vi "Stereo - Calibration Manager.vi"(7 "Function":T5, 10 "Right Grid Image":cluster{"Grid Image":T1, "Reference Points":T3}, 11 "Left Grid Image":cluster{"Grid Image":T1, "Reference Points":T3}) -> (0 "Calibration OK":bool, 1 "Calibrated Images":T1[](array[typedef]), 2 "Grid Coverage":T2, 3 "Grid Images out":cluster{"Left Image":T1, "Right Image":T1}[](array[cluster]))   [LabVIEW 2019]
doc: "Keeps track of the calibration grids needed to calibrate each camera.\nComputes the left and right camera models needed to compute the stereo calibration."
uses:
  Stereo - Calibration Manager Function.ctl
  <vilib>/vision/Image Controls.llb/IMAQ Image.ctl
  <vilib>/vision/Calibration.llb/Calibration Reference Points.ctl
  <vilib>/vision/Image Controls.llb/Vision Info Type2.ctl
  <vilib>/vision/NI_Vision_Development_Module.lvlib
panel:
  # "Overview: Keeps track of the calibration grids needed to calibrate each camera.\n                    Computes the left and right camera models needed to compute the stereo calibration."
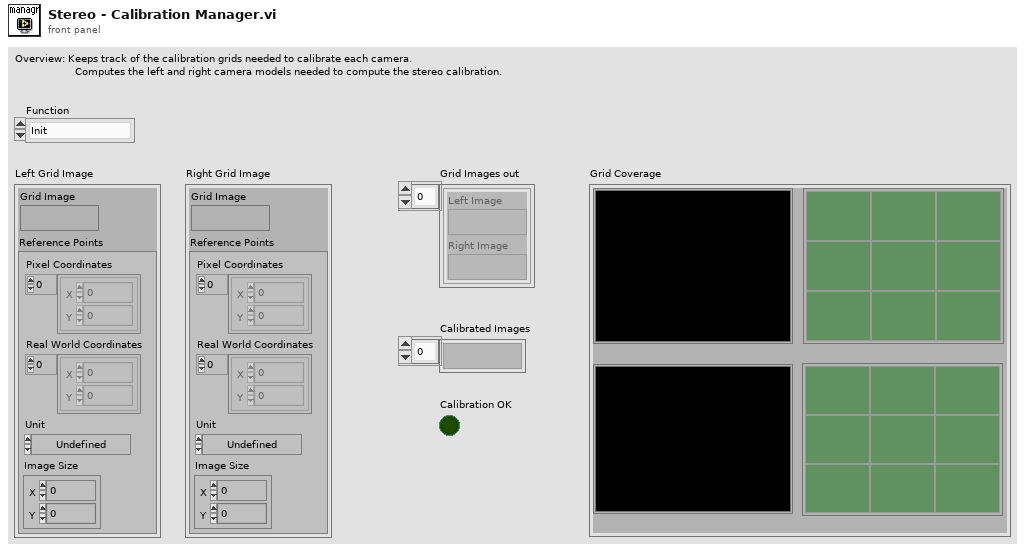
[diagram p1: front panel]
types:
  T1 = typedef "IMAQ Image.ctl" = refnum<image>
  T2 = cluster{"Left Image":T1, "Left Grid Coverage":bool[][], "Left Grid Coverage 3":string[][], "Right Image":T1, "Left Grid Coverage 2":bool[][], "Left Grid Coverage 4":string[][]}
  T3 = typedef "Calibration Reference Points.ctl" = cluster{"Pixel Coordinates":cluster{"X":dbl, "Y":dbl}[], "Real World Coordinates":cluster{"X":dbl, "Y":dbl}[], "Unit":T4, "Image Size":cluster{"X":u32, "Y":u32}}
  T4 = typedef "Image Unit" = enum32{"Undefined", "Angström", "Micrometer", "Millimeter", "Centimeter", "Meter", "Kilometer", "Microinch", "Inch", "Feet", "Nautical miles", "Standard miles", "Steps"}
  T5 = typedef "Stereo - Calibration Manager Function.ctl" = enum16{"Init", "Add Grid Images", "Get Images", "Dispose"}
  T6 = cluster{"Image Dst Out":T1, "Reference Points":T3}[][]
  T7 = cluster{"Left Image":T1, "Left Quadrants Status":bool[][], "Left Grid Coverage":string[][], "Right Image":T1, "Right Quadrant Status":bool[][], "Right Grid Coverage":string[][]}
  T8 = typedef "Vision Info Type2.ctl" = u32
  T9 = cluster{"Grid Image":T1, "Reference Points":T3}[]
  T10 = cluster{"Image Dst Out":T1, "Reference Points":T3}[]
  T11 = cluster{"Image Dst Out":T1, "Reference Points":T3}
  T12 = cluster{"Grid Image":T1, "Reference Points":T3}[][]
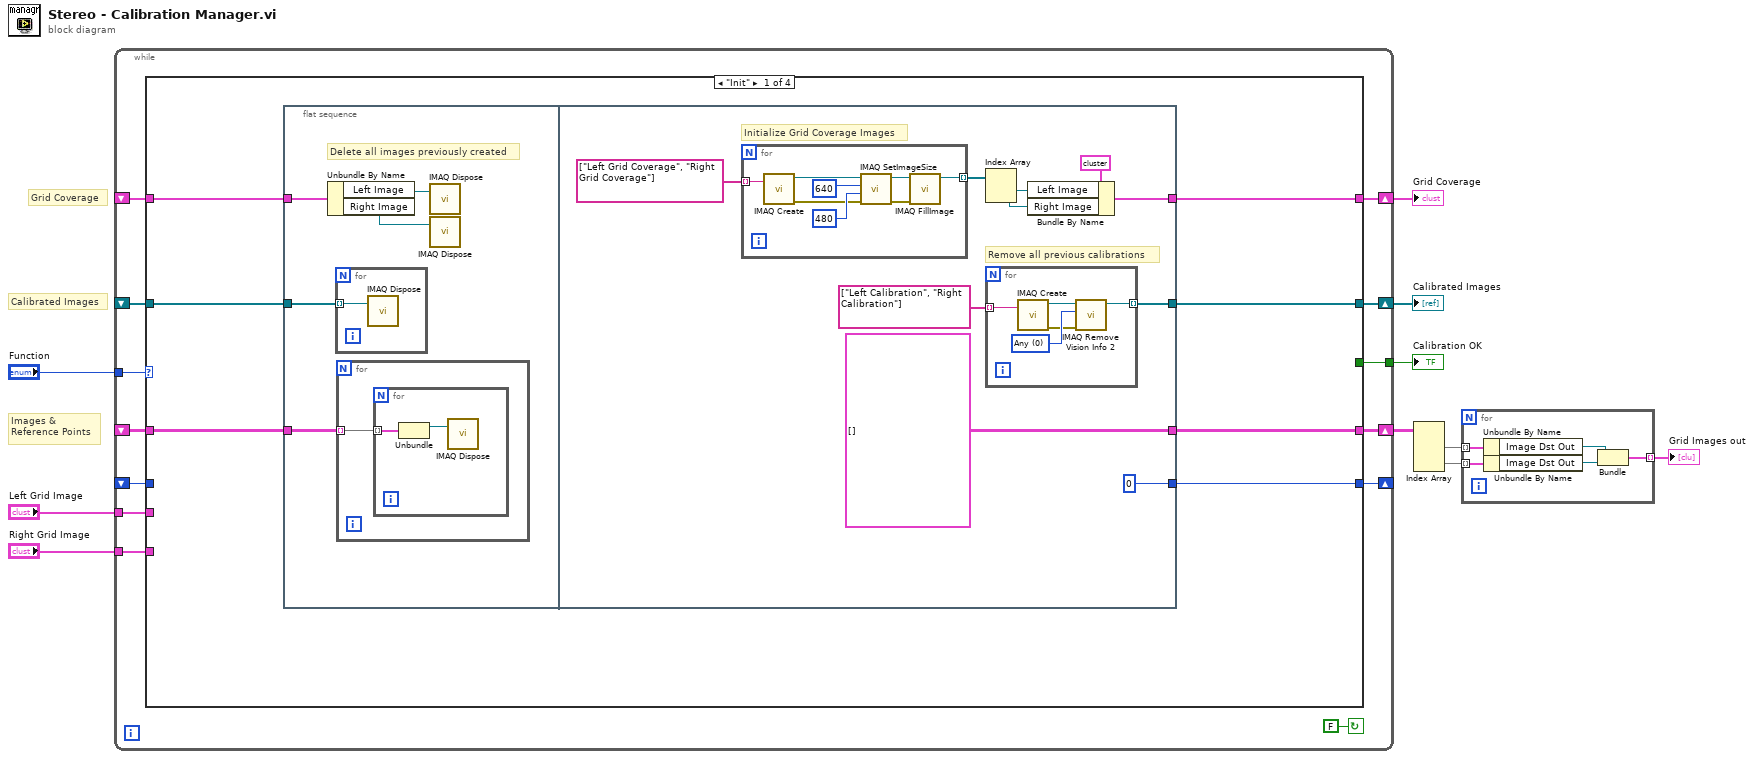
[diagram p0: block diagram]
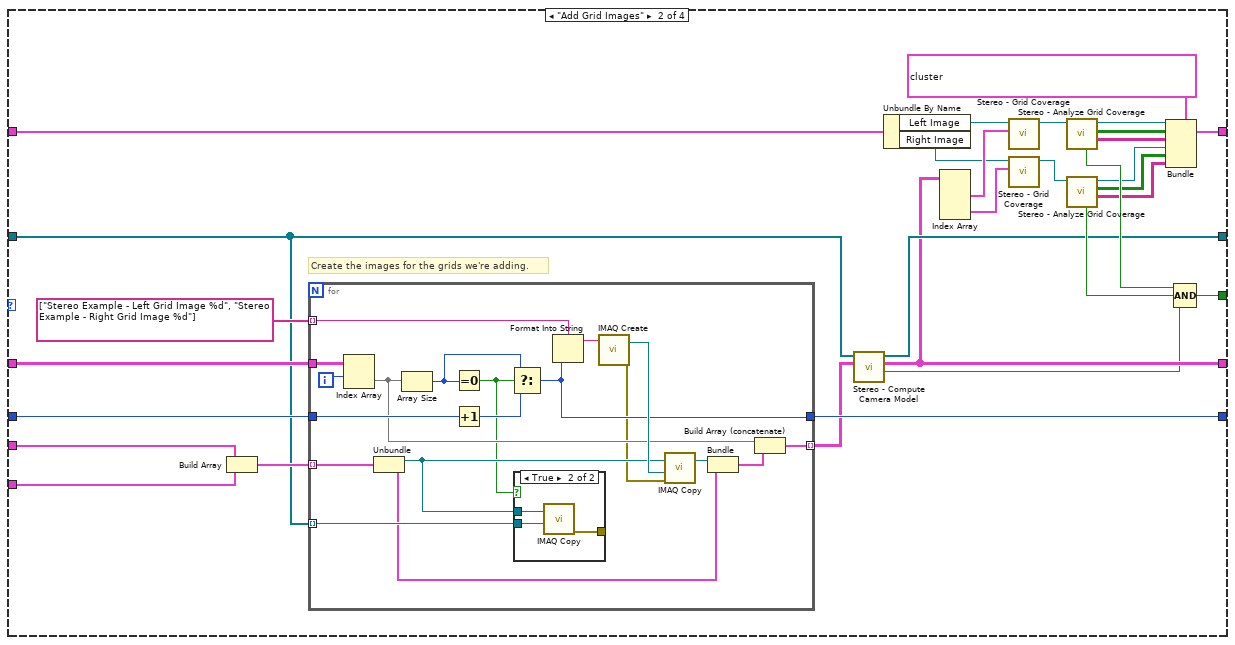
[diagram p2: hidden frame]
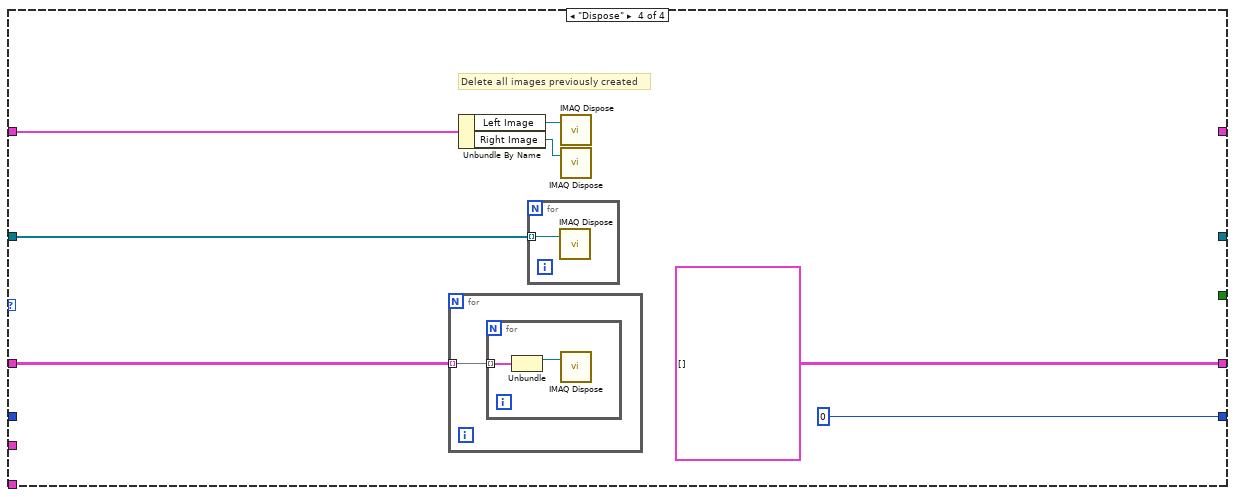
[diagram p5: hidden frame]
diagram:
  # "Calibrated Images"
  # "Grid Coverage"
  # "Images &\nReference Points"
  n1 = while {
    shift-right: [w23] -> w10
    shift-left: _ -> [w22]
    shift-right: [w19] -> w8
    shift-left: _ -> [w20]
    shift-right: [w17] -> _
    shift-left: _ -> [w18]
    shift-right: [w15] -> w5
    shift-left: _ -> [w16]
    tunnel: "Left Grid Image" -> [w14]
    tunnel: "Right Grid Image" -> [w13]
    tunnel: "Function" -> [w12]
    tunnel: [w11] -> w1
    stop <- FALSE continue-if-true
    n2 = case shown="\"Init\"" w12 {
      tunnel: [w30 w65 w117 _] -> w23
      tunnel: w22 -> [w25 w67 w117 w122]
      tunnel: w20 -> [w24 w92 w118 w125]
      tunnel: [w29 w64 w118 T6 []] -> w19
      tunnel: w18 -> [_ w91 w116 _]
      tunnel: [w28 w90 w116 0] -> w17
      tunnel: w16 -> [w26 w88 w115 w121]
      tunnel: [w27 w89 w115 _] -> w15
      tunnel: w14 -> [_ w87 _ _]
      tunnel: w13 -> [_ w86 _ _]
      tunnel: [_ w68 _ _] -> w11
      frame "Init" {
        n3 = flat-sequence {
          tunnel: w26 -> [w33]
          tunnel: w25 -> [w32]
          tunnel: w24 -> [w31]
          tunnel: [w49] -> w30
          tunnel: [T6 []] -> w29
          tunnel: [0] -> w28
          tunnel: [w46] -> w27
          frame #0 {
            # "Delete all images previously created"
            n4 = Unbundle By Name(w33) -> ("Left Image"=w34:T1, "Right Image"=w35:T1)
            n5 = for {
              tunnel: w32 -> [w36] mode=indexing
              n6 = call "IMAQ Dispose"("Image"=w36) -> ()  [unwired: 2 in, 4 out]
            }
            n7 = for {
              tunnel: w31 -> [w37] mode=indexing
              n8 = for {
                tunnel: w37 -> [w39] mode=indexing
                n9 = Unbundle(w39) -> ("Image Dst Out"=w38:T1)  [unwired: 1 out]
                n10 = call "IMAQ Dispose"("Image"=w38) -> ()  [unwired: 2 in, 4 out]
              }
            }
            n11 = call "IMAQ Dispose"("Image"=w34) -> ()  [unwired: 2 in, 4 out]
            n12 = call "IMAQ Dispose"("Image"=w35) -> ()  [unwired: 2 in, 4 out]
          }
          frame #1 {
            # "Remove all previous calibrations"
            # "Initialize Grid Coverage Images"
            n13 = for {
              tunnel: string[] ["Left Grid Coverage", "Right Grid Coverage"] -> [w55] mode=indexing
              tunnel: [w54] -> w43 mode=indexing
              n14 = call "IMAQ Create"("Image Name"=w55) -> ("New Image"=w57:T1, "error out"=w50:errorcluster)  [unwired: 3 in, 1 out]
              n15 = call "IMAQ SetImageSize"("error in (no error)"=w50, "Y Resolution"=480 ("X Resolution"), "X Resolution"=640, "Image"=w57) -> ("error out"=w51:errorcluster, "Image Out"=w56:T1)  [unwired: 1 out]
              n16 = call "IMAQ FillImage"("error in (no error)"=w51, "Image"=w56) -> ("Image Out"=w54:T1)  [unwired: 5 in, 4 out]
            }
            n17 = Index Array(array=w43) -> (element #1=w41:T1, element #2=w40:T1)  [unwired: 2 in]
            n18 = for {
              tunnel: string[] ["Left Calibration", "Right Calibration"] -> [w62] mode=indexing
              tunnel: [w59] -> w49 mode=indexing
              w60 = T8 0 items=["Any", "Calibration", "Overlay", "Grayscale Template", "Color Template", "Geometric Template", "Custom Data", "Golden Template", "Geometric Template 2", "Contour Data", "Camera Model"] ("Vision Info")
              n19 = call "IMAQ Create"("Image Name"=w62) -> ("New Image"=w61:T1, "error out"=w58:errorcluster)  [unwired: 3 in, 1 out]
              n20 = call "IMAQ Remove Vision Info 2"("error in (no error)"=w58, "Vision Info"=w60, "Image"=w61) -> ("Image Out"=w59:T1)  [unwired: 8 out]
            }
            n21 = Bundle By Name(cluster=T7 {"Left Image"=refnum, "Left Quadrants Status"=[], "Left Grid Coverage"=[], "Right Image"=refnum, "Right Quadrant Status"=[], "Right Grid Coverage"=[]} ("Grid Coverage 2"), "Left Image"=w41, "Right Image"=w40) -> (w46:T7)
          }
        }
      }
      frame "Add Grid Images" {
        # "Create the images for the grids we're adding."
        n22 = Build Array(w87, w86) -> (w70:T9)
        n23 = for {
          tunnel: w91 -> [w107]
          tunnel: [w106] -> w90
          tunnel: w67 -> [w103] mode=indexing
          tunnel: w70 -> [w102] mode=indexing
          tunnel: string[] ["Stereo Example - Left Grid Image %d", "Stereo Example - Right Grid Image %d"] -> [w100] mode=indexing
          tunnel: w92 -> [w97]
          tunnel: [w95] -> w66 mode=indexing
          i -> [w96]
          n24 = Index Array(array=w97, index (row)=w96) -> (element=w98:T10)  [unwired: 1 in]
          n25 = Unbundle(w102) -> ("Grid Image"=w101:T1, "Reference Points"=w99:T3)
          n26 = Array Size(array=w98) -> (size(s)=w108:i32)
          n27 = Equal To 0?(x=w108) -> (x = 0?=w94:bool)
          n28 = Increment(x=w107) -> (x+1=w109:i32)
          n29 = Select(t=w108, s=w94, f=w109) -> (s? t:f=w106:i32)
          n30 = case shown="True" w94 {
            tunnel: w103 -> [_ w114]
            tunnel: w101 -> [_ w113]
            tunnel: [_ w112] -> _
            frame False {
            }
            frame True {
              n31 = call "IMAQ Copy"("Image Dst"=w114, "Image Src"=w113) -> ("error out"=w112:errorcluster)  [unwired: 1 in, 4 out]
            }
          }
          n32 = Format Into String(format string=w100, w106) -> (resulting string=w110:string)  [unwired: 2 in, 1 out]
          n33 = call "IMAQ Create"("Image Name"=w110) -> ("New Image"=w111:T1, "error out"=w93:errorcluster)  [unwired: 3 in, 1 out]
          n34 = call "IMAQ Copy"("error in (no error)"=w93, "Image Dst"=w111, "Image Src"=w101) -> ("Image Dst Out"=w105:T1)  [unwired: 4 out]
          n35 = Bundle("Image Dst Out"=w105, "Reference Points"=w99) -> (w104:T11)  [unwired: 1 out]
          n36 = Build Array (concatenate)(w98, w104) -> (w95:T10)
        }
        n37 = call "Stereo - Compute Camera Model.vi"("Images and Reference Points in"=w66, "Images"=w67) -> ("Boolean"=w63:bool, "Images and Reference Points out"=w64:T12, "Calibrated Images"=w65:T1[])  [unwired: 7 in]
        n38 = Unbundle By Name(w88) -> ("Left Image"=w77:T1, "Right Image"=w76:T1)
        n39 = Index Array(array=w64) -> (element #1=w85:T9, element #2=w84:T9)  [unwired: 4 in]
        n40 = call "Stereo - Grid Coverage.vi"("Grid Images"=w85, "Image in"=w77) -> ("Image out"=w83:T1)  [unwired: 1 in, 8 out]
        n41 = call "Stereo - Grid Coverage.vi"("Grid Images"=w84, "Image in"=w76) -> ("Image out"=w82:T1)  [unwired: 1 in, 8 out]
        n42 = call "Stereo - Analyze Grid Coverage.vi"("Grid Coverage"=w83) -> ("Coverage %"=w74:string[][], "Quadrants OK"=w75:bool[][], "Grid Coverage (dup)"=w81:T1, "Coverage OK"=w79:bool)  [unwired: 3 in, 4 out]
        n43 = call "Stereo - Analyze Grid Coverage.vi"("Grid Coverage"=w82) -> ("Coverage %"=w72:string[][], "Quadrants OK"=w73:bool[][], "Grid Coverage (dup)"=w78:T1, "Coverage OK"=w80:bool)  [unwired: 3 in, 4 out]
        n44 = Bundle(cluster=T7 {"Left Image"=refnum, "Left Quadrants Status"=[], "Left Grid Coverage"=[], "Right Image"=refnum, "Right Quadrant Status"=[], "Right Grid Coverage"=[]} ("Grid Coverage 2"), "Left Image"=w81, "Left Quadrants Status"=w75, "Left Grid Coverage"=w74, "Right Image"=w78, "Right Quadrant Status"=w73, "Right Grid Coverage"=w72) -> (w89:T7)
        n45 = Compound Arithmetic op=AND(w79, w80, w63) -> (w68:bool)
      }
      frame "Get Images" {
      }
      frame "Dispose" {
        # "Delete all images previously created"
        n46 = for {
          tunnel: w125 -> [w127] mode=indexing
          n47 = for {
            tunnel: w127 -> [w129] mode=indexing
            n48 = Unbundle(w129) -> ("Image Dst Out"=w128:T1)  [unwired: 1 out]
            n49 = call "IMAQ Dispose"("Image"=w128) -> ()  [unwired: 2 in, 4 out]
          }
        }
        n50 = Unbundle By Name(w121) -> ("Left Image"=w120:T1, "Right Image"=w119:T1)
        n51 = for {
          tunnel: w122 -> [w126] mode=indexing
          n52 = call "IMAQ Dispose"("Image"=w126) -> ()  [unwired: 2 in, 4 out]
        }
        n53 = call "IMAQ Dispose"("Image"=w120) -> ()  [unwired: 2 in, 4 out]
        n54 = call "IMAQ Dispose"("Image"=w119) -> ()  [unwired: 2 in, 4 out]
      }
    }
  }
  "Calibrated Images" <- w10
  "Grid Coverage" <- w5
  "Calibration OK" <- w1
  n55 = Index Array(array=w8) -> (element #1=w7:T10, element #2=w6:T10)  [unwired: 4 in]
  n56 = for {
    tunnel: [w132] -> w9 mode=indexing
    tunnel: w7 -> [w131] mode=indexing
    tunnel: w6 -> [w130] mode=indexing
    n57 = Unbundle By Name(w131) -> ("Image Dst Out"=w134:T1)
    n58 = Unbundle By Name(w130) -> ("Image Dst Out"=w133:T1)
    n59 = Bundle("Image Dst Out"=w134, "Image Dst Out"=w133) -> (w132:cluster{"Image Dst Out":T1, "Image Dst Out":T1})  [unwired: 1 out]
  }
  "Grid Images out" <- w9
